vi "mean_fifo.vi"(8 "reset":bool, 11 "zk":fxp<+/-,16,5>) -> (0 "fifo_data":fxp<+/-,16,5>, 2 "mean":fxp<+/-,33,22>)   [LabVIEW 2017]
uses:
  <vilib>/Platform/TimedLoop/XDataNode/timing_clust.ctl
  <vilib>/Platform/TimedLoop/XDataNode/nitl_modes.ctl
  <vilib>/Platform/TimedLoop/XDataNode/wakeup.ctl
  <vilib>/rvi/IPIntegrationNode/IPINode_Typedef/niFpgaIPINodeSupportedFamilies.ctl
  <vilib>/rvi/Emulation/niFpgaEmulationIsFPGAContextNoSignature.vi
  <vilib>/rvi/FIFO/Fifo_Resource/nirvififoEmulationSetSize.vi
  <vilib>/rvi/DataTransferAndStorage/Container/Common/niFpgaContainerGetUniqueNameForEmu.vi
  <vilib>/rvi/FIFO/Fifo_Resource/nirviFifoEmulationQueueMgr.vi
  <instcachedir>/0/nirviFifoEmulationQueueMgr_E5CAEC123FF24DC58D834DCA3CDAA9B5.lvgen/nirviFifoEmulationQueueMgr_E5CAEC123FF24DC58D834DCA3CDAA9B5_001.vi
  <vilib>/rvi/Emulation/niFpgaProcessEmulError.vi
  <vilib>/rvi/Emulation/niFpgaSctlEmulationGetInTimedLoop.vi
  <vilib>/rvi/Emulation/niFpgaEmulationReportErrorSimple.vi
  <vilib>/rvi/Emulation/niFpgaGetClockAttributes.vi
  <vilib>/rvi/Emulation/niFpgaCriticalErrorInLSC.vi
  <vilib>/rvi/errors/niFpgaSetErrorForExecOnDevCompSimple.vi
  <vilib>/rvi/eio/common/nirviEmuReportErrorAndStop.vi
  <vilib>/Utility/error.llb/Clear Errors.vi
  <vilib>/rvi/FIFO/Fifo_Resource/nirvififoEmulationCreateLock.vi
  <vilib>/rvi/FIFO/Fifo_Resource/nirvififoEmulationObtainLock.vi
  <vilib>/rvi/FIFO/Fifo_Resource/nirvififoEmulationReleaseLock.vi
  <vilib>/rvi/occurrence/nirviWaitOnOccurrenceBase.vi
  <vilib>/rvi/errors/nirviReportUnexpectedCaseInternalError.vi
  <vilib>/rvi/errors/nirviReportUnexpectedCaseInternalError (U32).vi
  <vilib>/rvi/IPIntegrationNode/IPINode_Utilities/niFpgaIPINodeSimCore.vi
  <vilib>/rvi/DataTransferAndStorage/Container/XNode/niFpgaContainer.xnode
  <vilib>/rvi/FIFO/Fifo_Resource/nirvififoEmulationClear.vi
  <vilib>/platform/TimedLoop/XDataNode/XDataNode.xnode
  <vilib>/rvi/FXPMathLib/FxpSub/XNode/nifxpmath_Sub.xnode
  <vilib>/rvi/FIFO/Fifo_Resource/nirvififoEmulationRead.vi
  <vilib>/rvi/XilinxIP/XIPIN_XNode/niFpgaXIPIN.xnode
  mean_of_mem/Accumulator/Accumulator_1C7944CBDE2C441789DF23E9BDB4C226.dll
  <vilib>/rvi/IPIntegrationNode/IPINode_Xnode/niFpgaIPINode.xnode
  <vilib>/Platform/TimedLoop/XDataNode/XDNodeRunTimeDep.lvlib
  <vilib>/rvi/FXPMathLib/sim/FxpSim.dll
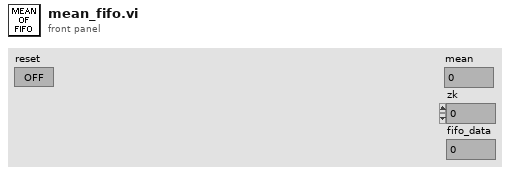
[diagram p1: front panel]
types:
  T1 = typedef "XDNodeRunTimeDep.lvlib/timing_clust.ctl" = cluster{"Expected End [f-1]":u64, "Actual End [f-1]":u64, "Finished Late? [f-1]":bool, "Expected End [i-1]":u64, "Actual End [i-1]":u64, "Finished Late? [i-1]":bool, "Expected Start [i]":u64, "Actual Start [i]":u64, "Expected Start [f]":u64, "Actual Start [f]":u64, "Source Name":string, "Structure Name":string, "Period":i64, "Deadline":i64, "Offset":i64, "Start":i64, "Priority":i32, "Timeout":i32, "Mode":T2, "Wakeup Reason":T3, "Error":errorcluster, "Source Type":string, "Secondary Source Type":string, "Global End Time":u64, "Global Start Time":u64, "Frame Duration":u64, "Iteration Duration":u64, "Assigned CPU":i32, "I/O Scan Engine Mode":u32}
  T2 = typedef "XDNodeRunTimeDep.lvlib/nitl_modes.ctl" = enum32{"No Change", "Process missed periods, maintain original phase", "Discard missed periods, maintain original phase", "Process missed periods, ignore original phase", "Discard missed periods, ignore original phase"}
  T3 = typedef "XDNodeRunTimeDep.lvlib/wakeup.ctl" = enum32{"Normal", "Aborted", "Asynchronous wakeup", "Timing source error", "Timed loop error", "Timeout"}
  T4 = typedef "niFpgaIPINodeSupportedFamilies.ctl" = cluster{"unlimited?":bool, "supported targets":string[]}
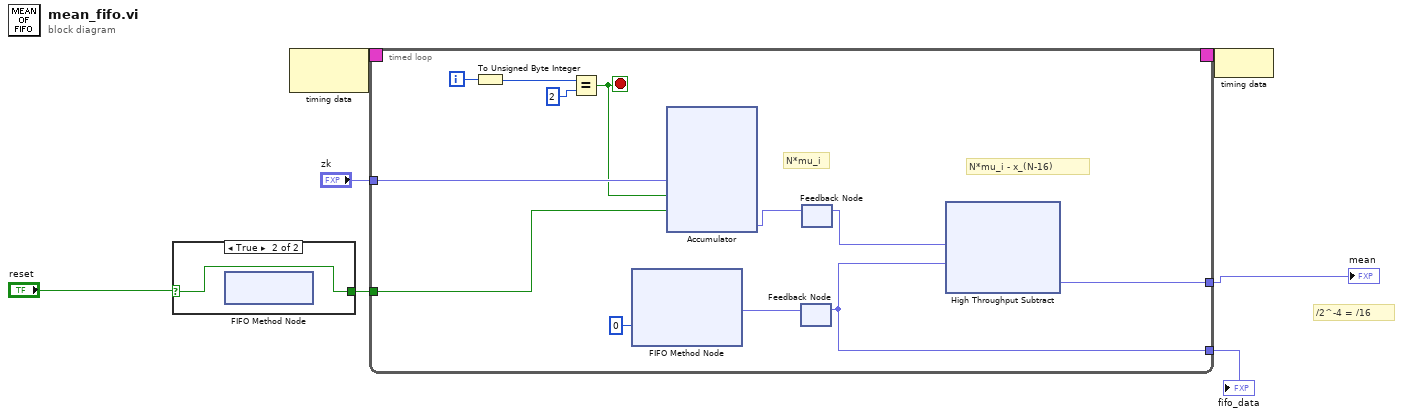
[diagram p0: block diagram]
diagram:
  # "/2^-4 = /16"
  n1 = case shown="True" "reset" {
    selector: "reset" -> [w8 w9]
    tunnel: [w8 w9] -> w3
    frame False {
    }
    frame True {
      n2 = xnode ("FIFO Method Node")() -> ()  [unwired: 1 in, 1 out]
    }
  }
  n3 = node-c288() -> (w7:T1)  [unwired: 1 in]
  n4 = timed-loop {
    timing: w7 -> [_]
    timing-out: [_] -> w6
    tunnel: "zk" -> [w21]
    tunnel: [w17] -> w1
    tunnel: w3 -> [w12]
    tunnel: [w11] -> w2
    i -> [w16]
    stop <- w10 stop-if-true
    # "N*mu_i - x_(N-16)"
    # "N*mu_i"
    n5 = To Unsigned Byte Integer(number=w16) -> (unsigned 8bit integer=w14:u8)
    n6 = Equal?(x=w14, y=u8 2) -> (x = y?=w10:bool)
    n7 = xnode ("FIFO Method Node")("Timeout"=0) -> ("Element"=w19:fxp<+/-,16,5>)  [unwired: 1 in, 2 out]
    n8 = xnode ("Accumulator")("b"=w21, "bypass"=w10, "sclr"=w12) -> ("q"=w20:fxp<+/-,32,21>)  [unwired: 1 in]
    n9 = feedback #1() -> (w11:fxp<+/-,16,5>)  [unwired: 1 in]
    n10 = feedback-in #1(w19) -> ()
    n11 = feedback-in #2(w20) -> ()
    n12 = feedback #2() -> (w18:fxp<+/-,32,21>)  [unwired: 1 in]
    n13 = xnode "High Throughput Subtract"("x"=w18, "y"=w11) -> ("x-y"=w17:fxp<+/-,33,22>)
  }
  "mean" <- w1
  "fifo_data" <- w2
  n14 = node-c288(w6) -> ()
